vi "ValveWriter.vi"(1 "Manual Valve States":T1) -> ()   [LabVIEW 2017]
uses:
  Controls/Manual Control.ctl
  <vilib>/rvi/eio/common/nirviEmuTemplateMethod_errors.vi
  <vilib>/eio/EIONode/EIONode.xnode
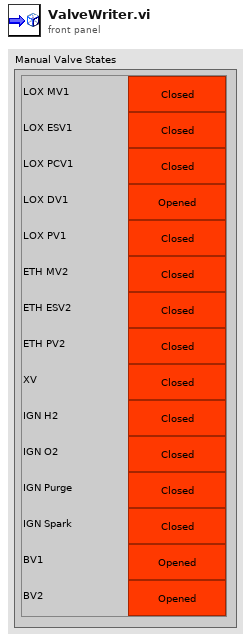
[diagram p1: front panel]
types:
  T1 = typedef "Manual Control.ctl" = cluster{"LOX MV1":bool, "LOX ESV1":bool, "LOX PCV1":bool, "LOX DV1":bool, "LOX PV1":bool, "ETH MV2":bool, "ETH ESV2":bool, "ETH PV2":bool, "XV":bool, "IGN H2":bool, "IGN O2":bool, "IGN Purge":bool, "IGN Spark":bool, "BV1":bool, "BV2":bool}
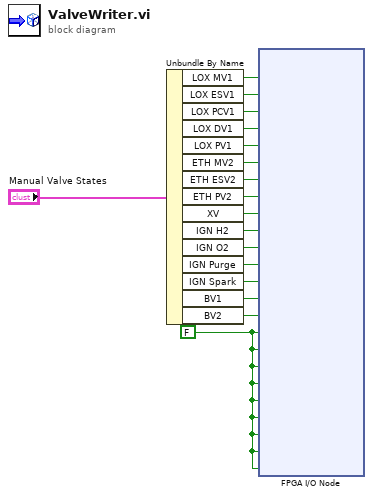
[diagram p0: block diagram]
diagram:
  w1 = FALSE ("DIDO/DO15")
  n1 = Unbundle By Name("Manual Valve States") -> ("LOX MV1"=w16:bool, "LOX ESV1"=w15:bool, "LOX PCV1"=w14:bool, "LOX DV1"=w13:bool, "LOX PV1"=w12:bool, "ETH MV2"=w11:bool, "ETH ESV2"=w10:bool, "ETH PV2"=w9:bool, "XV"=w2:bool, "IGN H2"=w3:bool, "IGN O2"=w8:bool, "IGN Purge"=w7:bool, "IGN Spark"=w6:bool, "BV1"=w5:bool, "BV2"=w4:bool)
  n2 = xnode "FPGA I/O Node"("DIDO/DO0"=w16, "DIDO/DO1"=w15, "DIDO/DO2"=w14, "DIDO/DO3"=w13, "DIDO/DO4"=w12, "DIDO/DO5"=w11, "DIDO/DO6"=w10, "DIDO/DO7"=w9, "DIDO/DO8"=w2, "DIDO/DO9"=w3, "DIDO/DO10"=w8, "DIDO/DO11"=w7, "DIDO/DO12"=w6, "DIDO/DO13"=w5, "DIDO/DO14"=w4, "DIDO/DO15"=w1, "PWM/DO0"=w1, "PWM/DO1"=w1, "PWM/DO2"=w1, "PWM/DO3"=w1, "PWM/DO4"=w1, "PWM/DO5"=w1, "PWM/DO6"=w1, "PWM/DO7"=w1) -> ()  [unwired: 24 in, 24 out]
